vi "Read Error Report.vi"(1 "Last Ack":refnum<class "Last Ack.lvclass">) -> (0 "error report":errorcluster)   [LabVIEW 2013, in "Actor Framework.lvlib" / "Last Ack.lvclass"]
doc: "(<B>Filename</B>: Actor Framework.lvlib:Last Ack.lvclass:Read Error Report.vi)\n\nReturns the error, if any, that caused an actor to shut down."
uses:
  <vilib>/ActorFramework/LastAck/Last Ack.lvclass
  <vilib>/ActorFramework/LastAck/Last Ack.lvclass/Last Ack.ctl
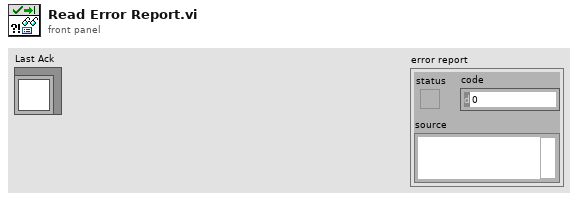
[diagram p1: front panel]
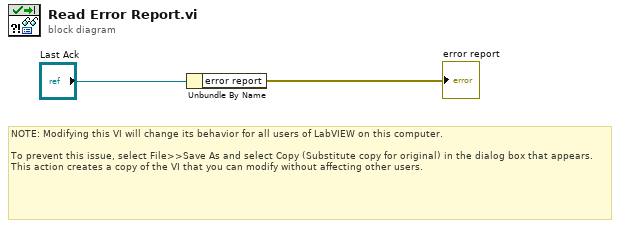
[diagram p0: block diagram]
diagram:
  # "NOTE: Modifying this VI will change its behavior for all users of LabVIEW on this computer.\n\nTo prevent this issue, select File>>Save As and select Copy (Substitute copy for original) in the dialog box that appears. This action creates a copy of the VI that you can modify without affecting other users."
  n1 = Unbundle By Name("Last Ack") -> ("error report"=→"error report":errorcluster)
